vi "ViTree.vi"   [LabVIEW 2014]
panel:
  # "Click CTRL + E\nTo View the Labspec VIs"
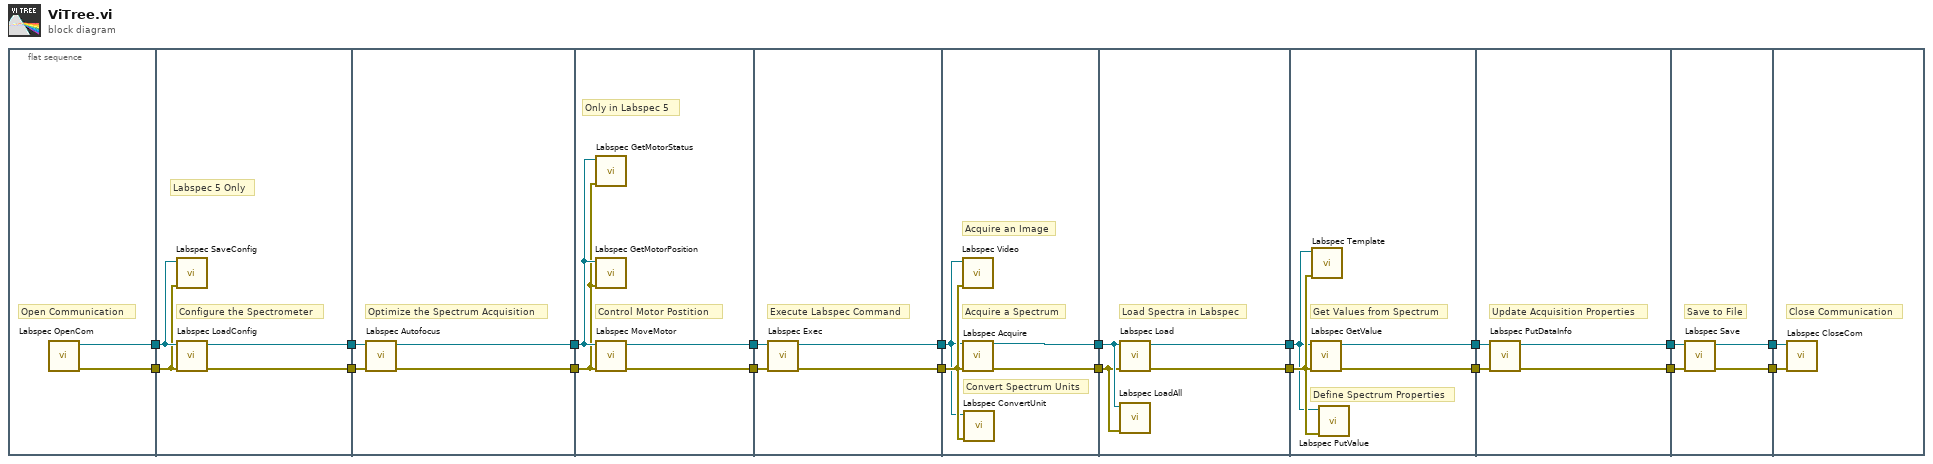
[diagram p0: block diagram]
diagram:
  n1 = flat-sequence {
    tunnel: [w22] -> w20
    tunnel: [w21] -> w19
    tunnel: w20 -> [w26]
    tunnel: w19 -> [w25]
    tunnel: [w24] -> w18
    tunnel: [w23] -> w17
    tunnel: w18 -> [w30]
    tunnel: w17 -> [w29]
    tunnel: [w28] -> w16
    tunnel: [w27] -> w15
    tunnel: w16 -> [w34]
    tunnel: w15 -> [w33]
    tunnel: [w32] -> w14
    tunnel: [w31] -> w13
    tunnel: w14 -> [w38]
    tunnel: w13 -> [w37]
    tunnel: [w36] -> w12
    tunnel: [w35] -> w11
    tunnel: w12 -> [w39]
    tunnel: w11 -> [w40]
    tunnel: [w42] -> w10
    tunnel: [w41] -> w9
    tunnel: w10 -> [w46]
    tunnel: w9 -> [w45]
    tunnel: [w44] -> w8
    tunnel: [w43] -> w7
    tunnel: w8 -> [w47]
    tunnel: w7 -> [w48]
    tunnel: [w50] -> w6
    tunnel: [w49] -> w5
    tunnel: w6 -> [w54]
    tunnel: w5 -> [w53]
    tunnel: [w52] -> w4
    tunnel: [w51] -> w3
    tunnel: w4 -> [w58]
    tunnel: w3 -> [w57]
    tunnel: [w56] -> w2
    tunnel: [w55] -> w1
    tunnel: w2 -> [w60]
    tunnel: w1 -> [w59]
    frame #0 {
      # "Open Communication"
      n2 = call "Labspec OpenCom.vi"() -> ("error out"=w21:errorcluster, "Automation Refnum"=w22:refnum<k7>)  [unwired: 1 in, 9 out]
    }
    frame #1 {
      # "Configure the Spectrometer"
      # "Labspec 5 Only"
      n3 = call "Labspec SaveConfig.vi"("error in"=w25, "Automation Refnum In"=w26) -> ()  [unwired: 2 in, 8 out]
      n4 = call "Labspec LoadConfig.vi"("error in"=w25, "Automation Refnum In"=w26) -> ("error out"=w23:errorcluster, "Automation Refnum Out"=w24:refnum<k7>)  [unwired: 2 in, 6 out]
    }
    frame #2 {
      # "Optimize the Spectrum Acquisition"
      n5 = call "Labspec Autofocus.vi"("error in"=w29, "Automation Refnum In"=w30) -> ("error out"=w27:errorcluster, "Automation Refnum Out"=w28:refnum<k7>)  [unwired: 8 out]
    }
    frame #3 {
      # "Only in Labspec 5"
      # "Control Motor Postition"
      n6 = call "Labspec GetMotorStatus.vi"("error in"=w33, "Automation Refnum In"=w34) -> ()  [unwired: 2 in, 7 out]
      n7 = call "Labspec GetMotorPosition.vi"("error in"=w33, "Automation Refnum In"=w34) -> ()  [unwired: 3 in, 7 out]
      n8 = call "Labspec MoveMotor.vi"("error in"=w33, "Automation Refnum In"=w34) -> ("error out"=w31:errorcluster, "Automation Refnum Out"=w32:refnum<k7>)  [unwired: 4 in, 4 out]
    }
    frame #4 {
      # "Execute Labspec Command"
      n9 = call "Labspec Exec.vi"("error in"=w37, "Automation Refnum In"=w38) -> ("error out"=w35:errorcluster, "Automation Refnum Out"=w36:refnum<k7>)  [unwired: 3 in, 5 out]
    }
    frame #5 {
      # "Convert Spectrum Units"
      # "Acquire an Image"
      # "Acquire a Spectrum"
      n10 = call "Labspec Video.vi"("error in"=w40, "Automation Refnum In"=w39) -> ()  [unwired: 1 in, 9 out]
      n11 = call "Labspec Acquire.vi"("Automation Refnum In"=w39, "error in"=w40) -> ("Automation Refnum Out"=w42:refnum<k7>, "error out"=w41:errorcluster)  [unwired: 10 in, 2 out]
      n12 = call "Labspec ConvertUnit.vi"("error in"=w40, "Automation Refnum In"=w39) -> ()  [unwired: 7 in, 3 out]
    }
    frame #6 {
      # "Load Spectra in Labspec"
      n13 = call "Labspec Load.vi"("error in"=w45, "Automation Refnum In"=w46) -> ("error out"=w43:errorcluster, "Automation Refnum Out"=w44:refnum<k7>)  [unwired: 1 in, 7 out]
      n14 = call "Labspec LoadAll.vi"("error in"=w45, "Automation Refnum In"=w46) -> ()  [unwired: 1 in, 9 out]
    }
    frame #7 {
      # "Define Spectrum Properties"
      # "Get Values from Spectrum"
      n15 = call "Labspec GetValue.vi"("error in"=w48, "Automation Refnum In"=w47) -> ("error out"=w49:errorcluster, "Automation Refnum Out"=w50:refnum<k7>)  [unwired: 3 in, 5 out]
      n16 = call "Labspec Template.vi"("error in"=w48, "Automation Refnum In"=w47) -> ()  [unwired: 7 in, 3 out]
      n17 = call "Labspec PutValue.vi"("error in"=w48, "Automation Refnum In"=w47) -> ()  [unwired: 3 in, 7 out]
    }
    frame #8 {
      # "Update Acquisition Properties"
      n18 = call "Labspec PutDataInfo.vi"("error in"=w53, "Automation Refnum In"=w54) -> ("error out"=w51:errorcluster, "Automation Refnum Out"=w52:refnum<k7>)  [unwired: 4 in, 4 out]
    }
    frame #9 {
      # "Save to File"
      n19 = call "Labspec Save.vi"("error in"=w57, "Automation Refnum In"=w58) -> ("error out"=w55:errorcluster, "Automation Refnum Out"=w56:refnum<k7>)  [unwired: 4 in, 4 out]
    }
    frame #10 {
      # "Close Communication"
      n20 = call "Labspec CloseCom.vi"("error in"=w59, "Automation Refnum In"=w60) -> ()  [unwired: 9 in, 1 out]
    }
  }
